vi "Statistique.vi"(10 "Waveform":waveform(dbl)) -> (1 "mean":dbl caption="moyenne" format="%0.2f", 2 "Valeur efficace":dbl, 3 "Fréquence":dbl)   [LabVIEW 2013]
uses:
  <vilib>/measure/matone.llb/Extract Single Tone Information 1 Chan.vi
  <vilib>/measure/NI_MAPro.lvlib
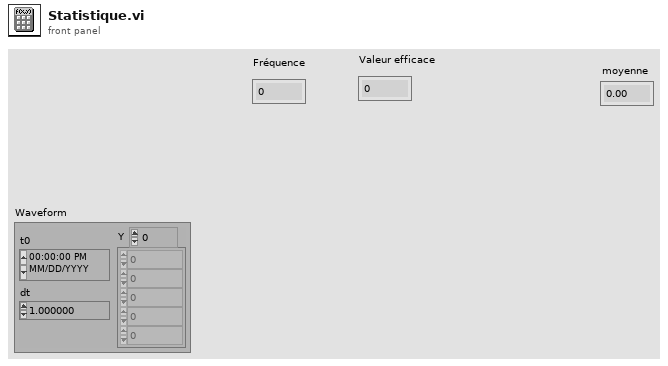
[diagram p1: front panel]
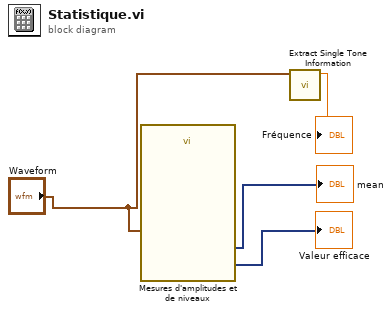
[diagram p0: block diagram]
diagram:
  n1 = call "Mesures d'amplitudes et de niveaux"("Signals"="Waveform") -> ("Mean (DC)"=→"mean":dynamicdata, "RMS"=→"Valeur efficace":dynamicdata)  [unwired: 12 in, 1 out]
  n2 = call-poly <vilib>:"Extract Single Tone Information.vi"("time signal in"="Waveform") -> ("detected frequency"=→"Fréquence":dbl)  [unwired: 5 in, 5 out]
